vi "Interrupt_1min.vi"() -> (2 "Boolean 2":bool)   [LabVIEW 2016]
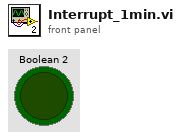
[diagram p1: front panel]
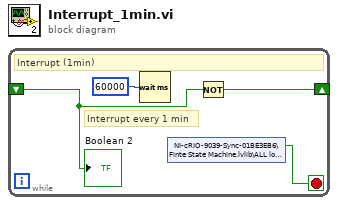
[diagram p0: block diagram]
diagram:
  n1 = while {
    shift-right: [w3] -> _
    shift-left: _ -> [w2]
    stop <- w1 stop-if-true
    # "Interrupt every 1 min"
    # "Interrupt (1min)"
    n2 = Wait (ms)(milliseconds to wait=u32 60000) -> ()  [unwired: 1 out]
    n3 = shared-variable "NI-cRIO-9039-Sync-01BE3EB6\\Finte State Machine.lvlib\\ALL loop stop"() -> (w1:bool)  [unwired: 1 in, 1 out]
    n4 = Not(x=w2) -> (.not. x?=w3:bool)
    "Boolean 2" <- w2
  }
